vi "TargetNew.vi"() -> ()   [LabVIEW 2018]
uses:
  <vilib>/Platform/TimedLoop/XDataNode/timing_clust.ctl
  <vilib>/Platform/TimedLoop/XDataNode/nitl_modes.ctl
  <vilib>/Platform/TimedLoop/XDataNode/wakeup.ctl
  <vilib>/rvi/eio/common/nirviEmuTemplateMethod_errors.vi
  <vilib>/rvi/Emulation/niFpgaGetClockAttributes.vi
  <vilib>/rvi/Emulation/niFpgaSctlEmulationGetInTimedLoop.vi
  <vilib>/rvi/Emulation/niFpgaEmulationReportErrorSimple.vi
  <vilib>/rvi/Emulation/niFpgaCriticalErrorInLSC.vi
  <vilib>/rvi/interface/RandomDataEmulation/niFpgaRandomDataHandleErrors.vi
  <vilib>/rvi/Emulation/niFpgaProcessEmulError.vi
  <vilib>/eio/EIONode/EIONode.xnode
  <vilib>/Platform/TimedLoop/XDataNode/XDataNode.xnode
  <vilib>/rvi/DataTransferAndStorage/Container/XNode/niFpgaContainer.xnode
  <vilib>/rvi/interface/RandomDataEmulation/nirviRandomDataFpgaReadWriteTemplate.vi
  <vilib>/Platform/TimedLoop/XDataNode/XDNodeRunTimeDep.lvlib
panel:
  out "MISO 3":bool[](array[boolean])
  in  "10 2":u8=10
  out "out 2":bool
  out "out 2":u8
  out "out":u8
  out "out":bool
  in  "10":u8=10
  out "MISO 2":bool[](array[boolean])
  in  "Такт CSN 18":u8=18
  in  "Такт CSN 26":u8=26
  in  "26_STOP":u8=26
  in  "18_STOP":u8=18
  in  "18_R":u8=17
  in  "26_R":u8=25
  in  "17":u8=17
  in  "25":u8=25
  in  "TRIG":bool
  in  "Сброс индикатора":bool
  out "SPI_is_done":bool
  in  "Делитель 24/x":u8=2
  in  "Автомат":bool
  in  "RESET":bool
  in  "MOSI":bool[](array[boolean])=[FALSE, FALSE, FALSE, FALSE, FALSE, FALSE, FALSE, FALSE, FALSE, FALSE, FALSE, FALSE, FALSE, FALSE, FALSE, FALSE, FALSE, FALSE, FALSE, FALSE, FALSE, FALSE, FALSE, FALSE]
  in  "SPI":bool
  in  "8-bit(F)/16-bit(T)":bool
  in  "Stop_FPGA":bool
  # "0"
  # "0"
  # "7"
  # "7"
  # "Начало слова (8 bit)"
  # "Конец адреса (8 bit)"
  # "8"
  # "Начало адреса (8 bit)"
  # "14"
  # "15"
  # "R(F)/W(T) (8 bit)"
  # "Начало слова (16 bit)"
  # "15"
  # "Конец адреса (16 bit)"
  # "16"
  # "Начало адреса (16 bit)"
  # "22"
  # "R(F)/W(T) (16 bit)"
  # "23"
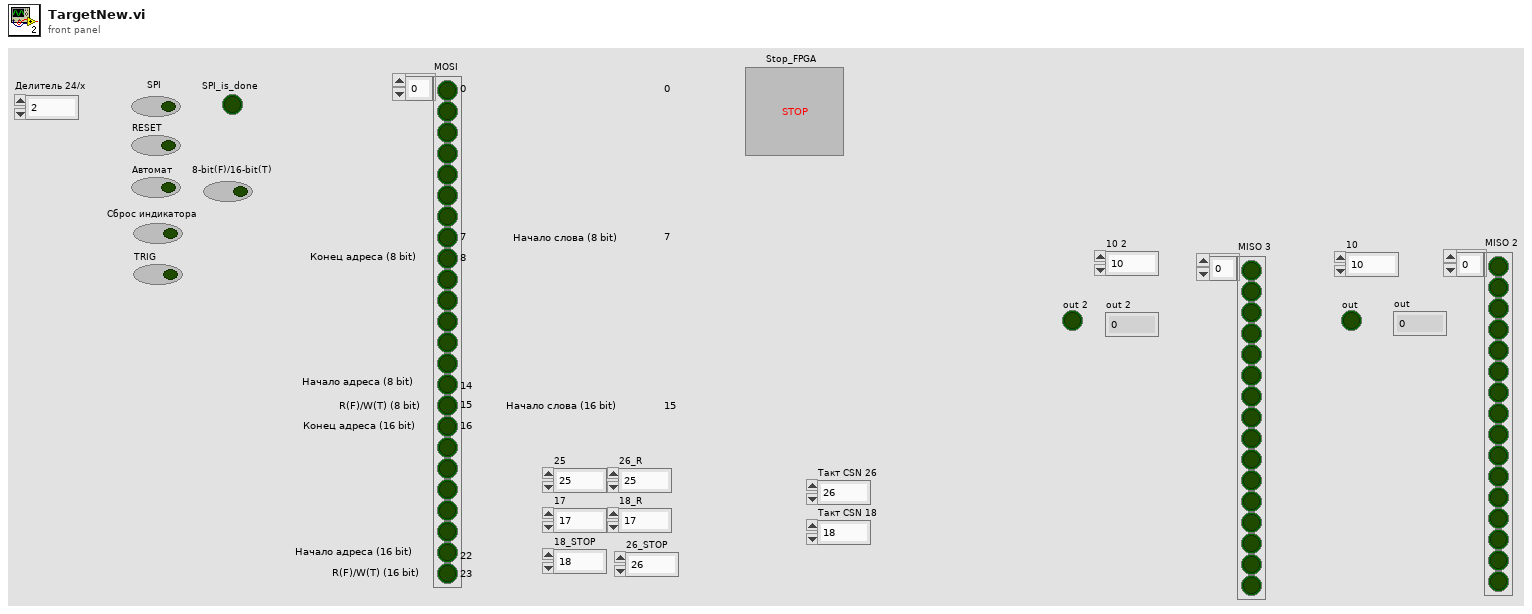
[diagram p1: front panel]
types:
  T1 = typedef "XDNodeRunTimeDep.lvlib/timing_clust.ctl" = cluster{"Expected End [f-1]":u64, "Actual End [f-1]":u64, "Finished Late? [f-1]":bool, "Expected End [i-1]":u64, "Actual End [i-1]":u64, "Finished Late? [i-1]":bool, "Expected Start [i]":u64, "Actual Start [i]":u64, "Expected Start [f]":u64, "Actual Start [f]":u64, "Source Name":string, "Structure Name":string, "Period":i64, "Deadline":i64, "Offset":i64, "Start":i64, "Priority":i32, "Timeout":i32, "Mode":T2, "Wakeup Reason":T3, "Error":errorcluster, "Source Type":string, "Secondary Source Type":string, "Global End Time":u64, "Global Start Time":u64, "Frame Duration":u64, "Iteration Duration":u64, "Assigned CPU":i32, "I/O Scan Engine Mode":u32}
  T2 = typedef "XDNodeRunTimeDep.lvlib/nitl_modes.ctl" = enum32{"No Change", "Process missed periods, maintain original phase", "Discard missed periods, maintain original phase", "Process missed periods, ignore original phase", "Discard missed periods, ignore original phase"}
  T3 = typedef "XDNodeRunTimeDep.lvlib/wakeup.ctl" = enum32{"Normal", "Aborted", "Asynchronous wakeup", "Timing source error", "Timed loop error", "Timeout"}
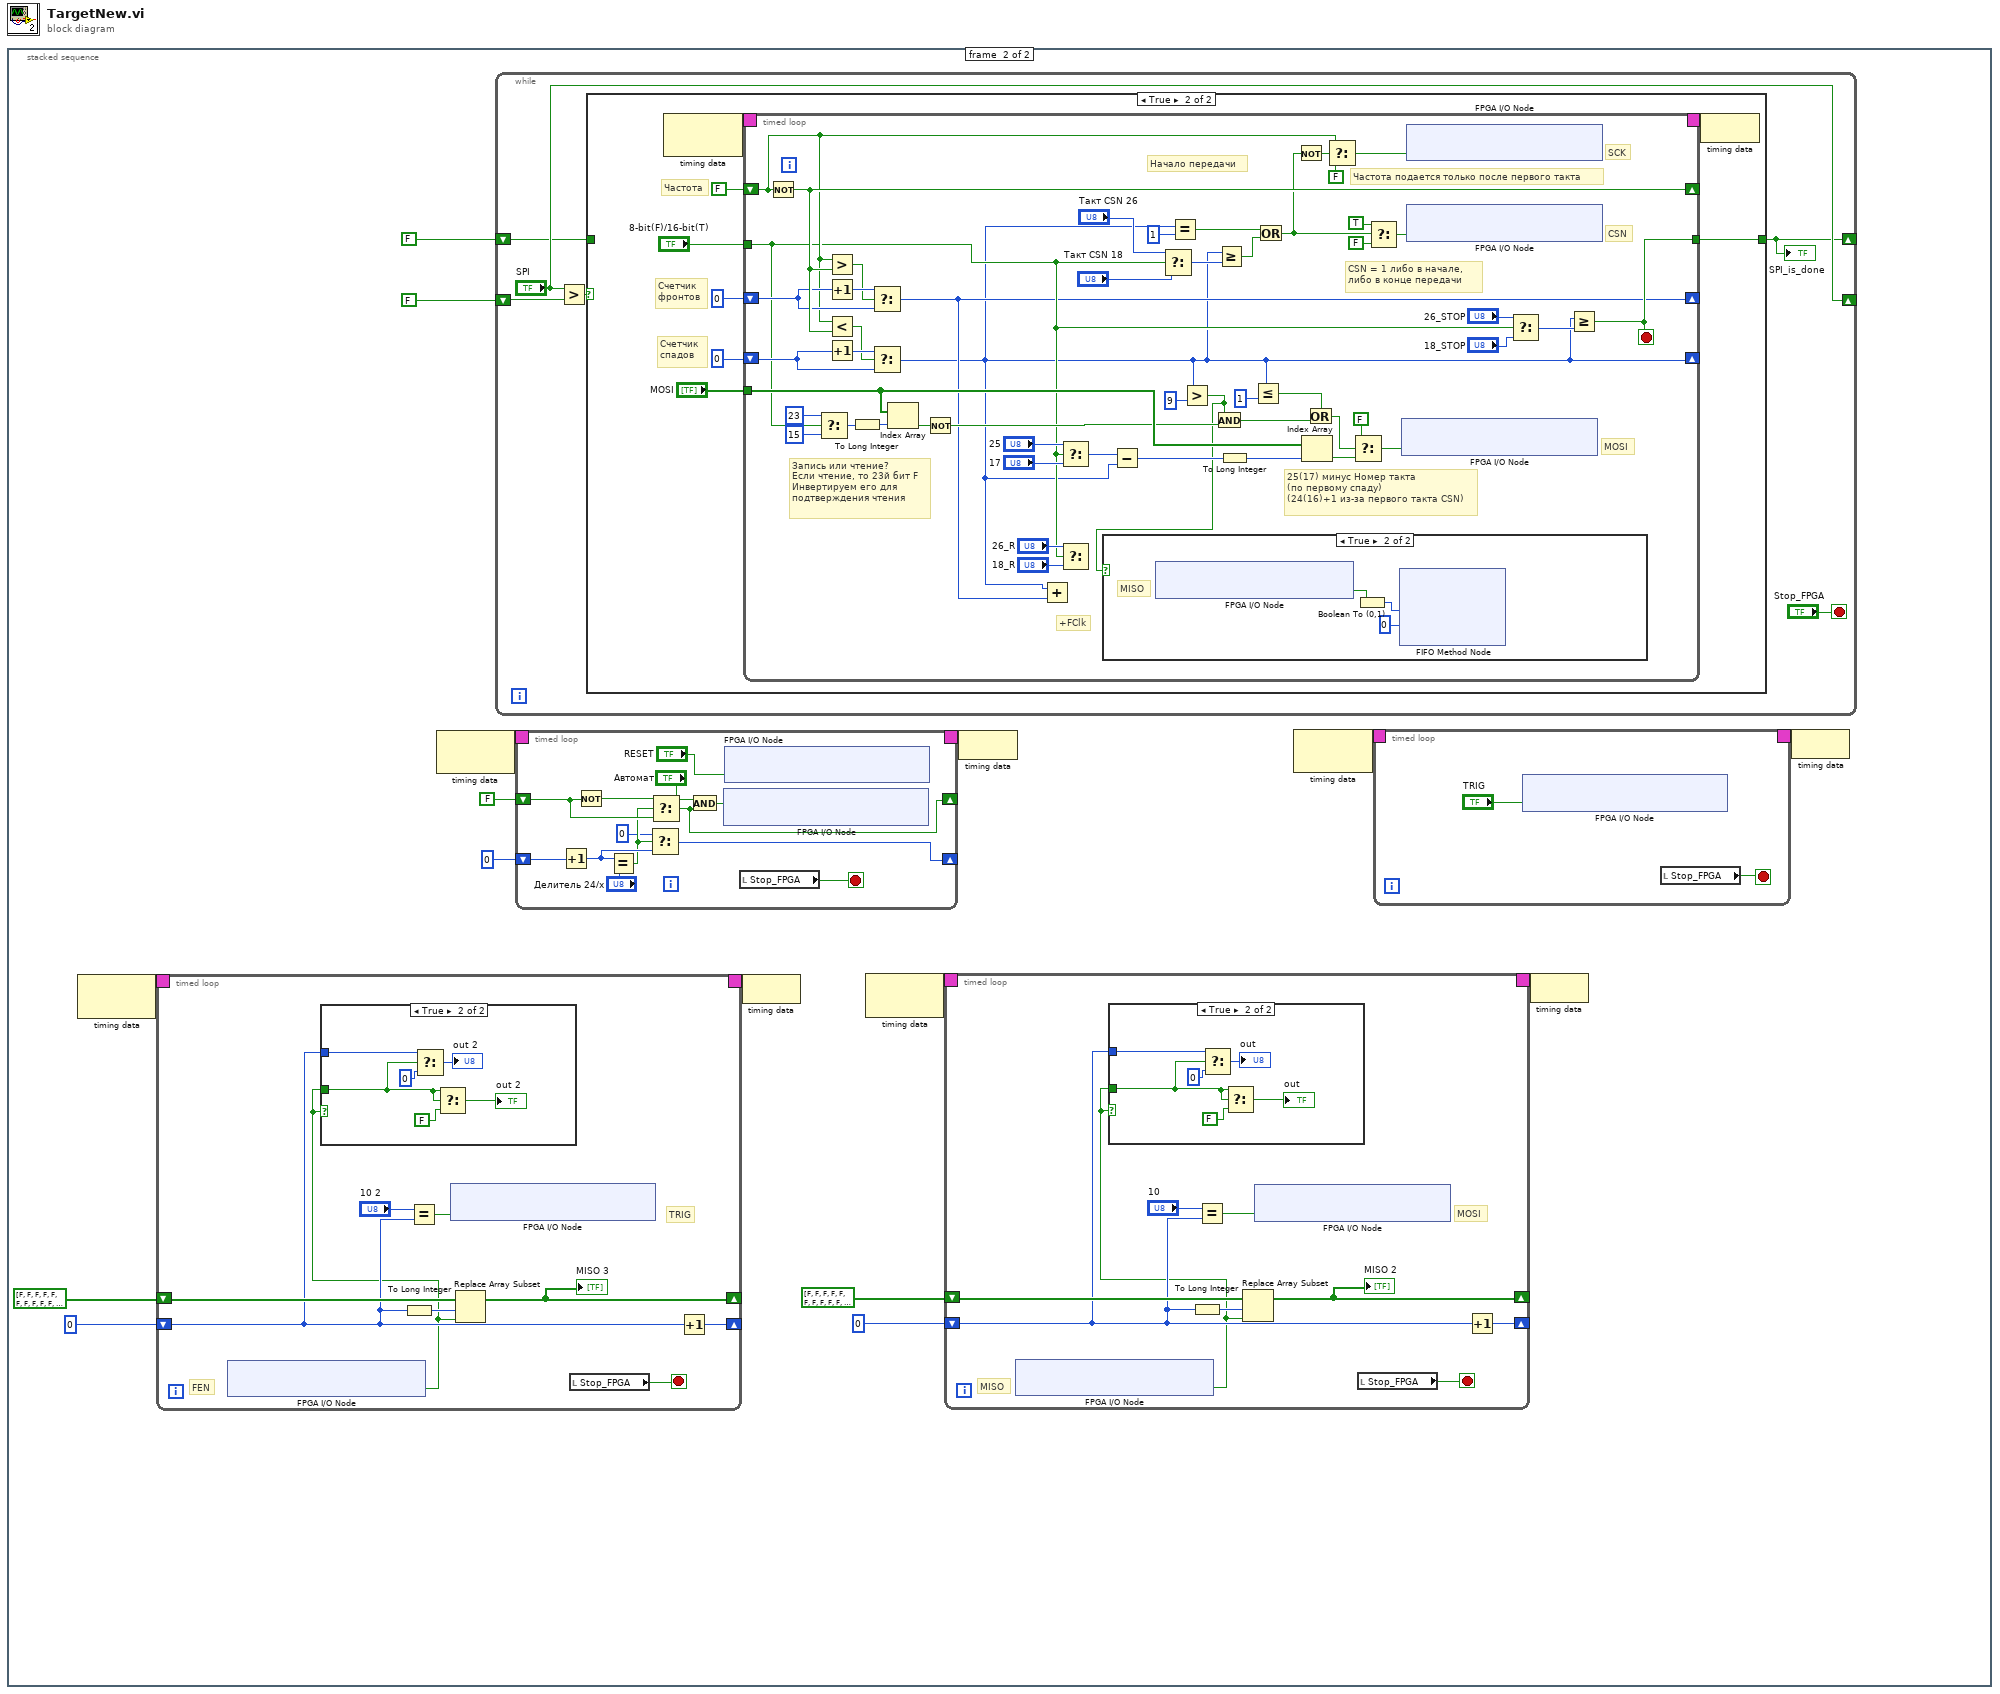
[diagram p0: block diagram]
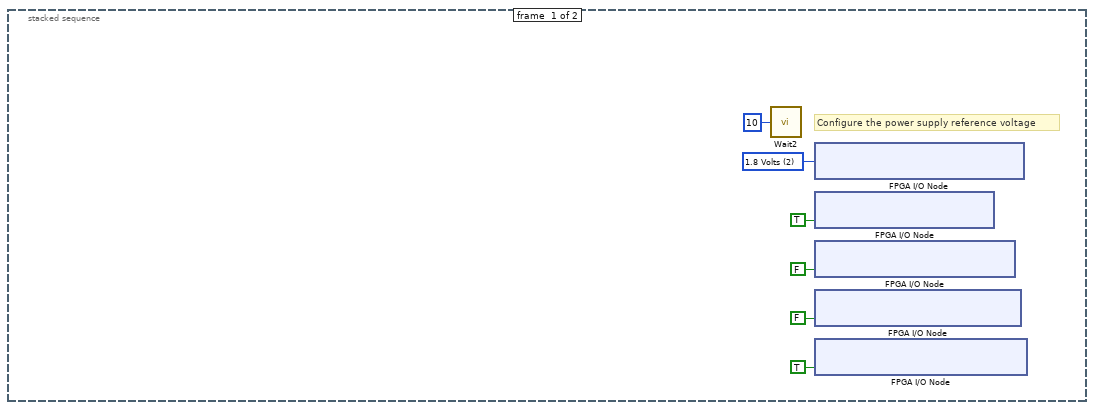
[diagram p2: hidden frame]
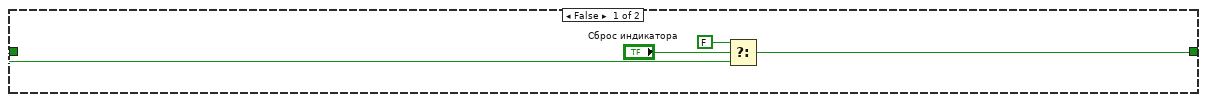
[diagram p5: hidden frame]
diagram:
  n1 = stacked-sequence {
    frame #0 {
      w6 = u8 2 items=["3.3 Volts", "2.5 Volts", "1.8 Volts"] ("Internal Power Supply Voltage")
      # "Configure the power supply reference voltage"
      n2 = call "Wait2"("Count(mSec)"=u8 10) -> ()  [unwired: 1 out]
      n3 = xnode "FPGA I/O Node"("IO Module\\Local_Supply_Select"=w6) -> ()  [unwired: 1 in, 1 out]
      n4 = xnode "FPGA I/O Node"("IO Module\\DDCA_PFI_WE"=TRUE ("IO Module\\DDCB_PFI_WE")) -> ()  [unwired: 1 in, 1 out]
      n5 = xnode "FPGA I/O Node"("IO Module\\DDCA_DIO0-7_WE"=FALSE ("IO Module\\DDCA_DIO0-7_WE")) -> ()  [unwired: 1 in, 1 out]
      n6 = xnode "FPGA I/O Node"("IO Module\\DDCA_DIO8-15_WE"=FALSE ("IO Module\\DDCA_DIO8-15_WE")) -> ()  [unwired: 1 in, 1 out]
      n7 = xnode "FPGA I/O Node"("IO Module\\DDCA_DIO16-23_WE"=TRUE ("IO Module\\DDCA_DIO16-23_WE")) -> ()  [unwired: 1 in, 1 out]
    }
    frame #1 {
      n8 = node-c288() -> (w10:T1)  [unwired: 1 in]
      n9 = timed-loop {
        timing: w10 -> [_]
        timing-out: [_] -> w9
        shift-right: [w30] -> _
        shift-left: bool[] [FALSE, FALSE, FALSE, FALSE, FALSE, FALSE, FALSE, FALSE, FALSE, FALSE, FALSE, FALSE, FALSE, FALSE, FALSE, FALSE] -> [w26]
        shift-right: [w27] -> _
        shift-left: u8 0 -> [w25]
        stop <- w28 stop-if-true
        # "FEN"
        # "TRIG"
        n10 = xnode "FPGA I/O Node"() -> ("IO Module\\DDCA_DIO1_Read"=w24:bool)  [unwired: 1 in, 1 out]
        n11 = case shown="True" w24 {
          tunnel: w25 -> [_ w33]
          tunnel: w24 -> [_ w32]
          frame False {
          }
          frame True {
            n12 = Select(t=w33, s=w32, f=u8 0) -> (s? t:f=→"out 2":u8)
            n13 = Select(t=w32, s=w32, f=FALSE ("t")) -> (s? t:f=→"out 2":bool)
          }
        }
        n14 = To Long Integer(number=w25) -> (32bit integer=w31:i32)
        n15 = Equal?(x="10 2", y=w25) -> (x = y?=w23:bool)
        n16 = xnode "FPGA I/O Node"("IO Module\\DDCA_DIO18_Write"=w23) -> ()  [unwired: 1 in, 1 out]
        n17 = Replace Array Subset(array=w26, new element=w24, index=w31) -> (w30:bool[])
        "MISO 3" <- w30
        n18 = local read "Stop_FPGA"() -> (w28:bool)
        n19 = Increment(x=w25) -> (x+1=w27:u8)
      }
      n20 = node-c288() -> (w21:T1)  [unwired: 1 in]
      n21 = while {
        shift-right: ["SPI"] -> _
        shift-left: FALSE -> [w89]
        shift-right: [w84] -> _
        shift-left: FALSE -> [w85]
        stop <- "Stop_FPGA" stop-if-true
        n22 = Greater?(x="SPI", y=w89) -> (0:w88:bool)
        n23 = case shown="True" w88 {
          tunnel: [w92 w96] -> w84
          tunnel: w85 -> [w90 _]
          frame False {
            n24 = Select(t=FALSE, s="Сброс индикатора", f=w90) -> (s? t:f=w92:bool)
          }
          frame True {
            # "Счетчик\nфронтов"
            # "Счетчик\nспадов"
            # "Частота"
            n25 = node-c288() -> (w101:T1)  [unwired: 1 in]
            n26 = timed-loop {
              timing: w101 -> [_]
              timing-out: [_] -> w100
              shift-right: [w105] -> _
              shift-left: u8 0 -> [w148]
              shift-right: [w151] -> _
              shift-left: FALSE -> [w142]
              shift-right: [w104] -> _
              shift-left: u8 0 -> [w149]
              tunnel: [w110] -> w96
              tunnel: "8-bit(F)/16-bit(T)" -> [w107]
              tunnel: "MOSI" -> [w129]
              stop <- w110 stop-if-true
              # "+FClk"
              # "MOSI"
              # "25(17) минус Номер такта\n(по первому спаду)\n(24(16)+1 из-за первого такта CSN)"
              # "Запись или чтение?\nЕсли чтение, то 23й бит F\nИнвертируем его для\nподтверждения чтения"
              # "Начало передачи"
              # "CSN"
              # "Частота подается только после первого такта"
              # "CSN = 1 либо в начале,\nлибо в конце передачи"
              # "SCK"
              n27 = Not(x=w142) -> (.not. x?=w151:bool)
              n28 = Select(t=u8 23, s=w107, f=u8 15) -> (s? t:f=w139:u8)
              n29 = Greater?(x=w142, y=w151) -> (0:w114:bool)
              n30 = Increment(x=w148) -> (x+1=w152:u8)
              n31 = Less?(x=w142, y=w151) -> (x < y?=w123:bool)
              n32 = Increment(x=w149) -> (x+1=w150:u8)
              n33 = To Long Integer(number=w139) -> (32bit integer=w138:i32)
              n34 = Select(t=w152, s=w114, f=w148) -> (s? t:f=w105:u8)
              n35 = Select(t=w150, s=w123, f=w149) -> (s? t:f=w104:u8)
              n36 = Index Array(array=w129, index=w138) -> (element=w124:bool)
              n37 = Not(x=w124) -> (.not. x?=w122:bool)
              n38 = Add(x=w104, y=w105) -> ()  [unwired: 1 out]
              n39 = Select(t="25", s=w107, f="17") -> (s? t:f=w119:u8)
              n40 = Select(t="26_R", s=w107, f="18_R") -> ()  [unwired: 1 out]
              n41 = Subtract(x=w119, y=w104) -> (x-y=w113:u8)
              n42 = Select(t="Такт CSN 26", s=w107, f="Такт CSN 18") -> (s? t:f=w118:u8)
              n43 = Equal?(x=w104, y=u8 1 ("1")) -> (x = y?=w144:bool)
              n44 = Greater?(x=w104, y=u8 9 ("18")) -> (0:w102:bool)
              n45 = case shown="True" w102 {
                frame False {
                }
                frame True {
                  # "MISO"
                  n46 = xnode "FPGA I/O Node"() -> ("IO Module\\DDCA_DIO0_Read"=w155:bool)  [unwired: 1 in, 1 out]
                  n47 = Boolean To (0,1)(Boolean=w155) -> (0, 1=w154:i16)
                  n48 = xnode ("FIFO Method Node")("Element"=w154, "Timeout"=0) -> ()  [unwired: 1 in, 2 out]
                }
              }
              n49 = And(x=w102, y=w122) -> (x .and. y?=w133:bool)
              n50 = Greater Or Equal?(x=w104, y=w118) -> (x >= y?=w115:bool)
              n51 = To Long Integer(number=w113) -> (32bit integer=w147:i32)
              n52 = Less Or Equal?(x=w104, y=u8 1 ("18")) -> (x <= y?=w131:bool)
              n53 = Or(x=w144, y=w115) -> (x .or. y?=w116:bool)
              n54 = Not(x=w116) -> (.not. x?=w117:bool)
              n55 = Index Array(array=w129, index=w147) -> (element=w137:bool)
              n56 = Or(x=w131, y=w133) -> (x .or. y?=w132:bool)
              n57 = Select(t=w142, s=w117, f=FALSE) -> (s? t:f=w143:bool)
              n58 = Select(t=FALSE, s=w132, f=w137) -> (s? t:f=w103:bool)
              n59 = Select(t=TRUE, s=w116, f=FALSE) -> (s? t:f=w135:bool)
              n60 = xnode "FPGA I/O Node"("IO Module\\DDCA_PFI3_Write"=w103) -> ()  [unwired: 1 in, 1 out]
              n61 = xnode "FPGA I/O Node"("IO Module\\DDCA_PFI1_Write"=w143) -> ()  [unwired: 1 in, 1 out]
              n62 = xnode "FPGA I/O Node"("IO Module\\DDCA_PFI2_Write"=w135) -> ()  [unwired: 1 in, 1 out]
              n63 = Select(t="26_STOP", s=w107, f="18_STOP") -> (s? t:f=w106:u8)
              n64 = Greater Or Equal?(x=w104, y=w106) -> (x >= y?=w110:bool)
            }
            n65 = node-c288(w100) -> ()
          }
        }
        "SPI_is_done" <- w84
      }
      n66 = timed-loop {
        timing: w21 -> [_]
        timing-out: [_] -> w20
        shift-right: [w68] -> _
        shift-left: FALSE -> [w77]
        shift-right: [w69] -> _
        shift-left: u8 0 -> [w74]
        stop <- w67 stop-if-true
        n67 = Increment(x=w74) -> (x+1=w72:u8)
        n68 = Not(x=w77) -> (.not. x?=w78:bool)
        n69 = Equal?(x=w72, y="Делитель 24/x") -> (x = y?=w71:bool)
        n70 = Select(t=u8 0, s=w71, f=w72) -> (s? t:f=w69:u8)
        n71 = Select(t=w78, s=w71, f=w77) -> (s? t:f=w68:bool)
        n72 = And(x="Автомат", y=w68) -> (x .and. y?=w76:bool)
        n73 = xnode "FPGA I/O Node"("IO Module\\DDCA_DIO16_Write"=w76) -> ()  [unwired: 1 in, 1 out]
        n74 = xnode "FPGA I/O Node"("IO Module\\DDCA_DIO19_Write"="RESET") -> ()  [unwired: 1 in, 1 out]
        n75 = local read "Stop_FPGA"() -> (w67:bool)
      }
      n76 = node-c288(w9) -> ()
      n77 = node-c288() -> (w14:T1)  [unwired: 1 in]
      n78 = timed-loop {
        timing: w14 -> [_]
        timing-out: [_] -> w13
        shift-right: [w49] -> _
        shift-left: bool[] [FALSE, FALSE, FALSE, FALSE, FALSE, FALSE, FALSE, FALSE, FALSE, FALSE, FALSE, FALSE, FALSE, FALSE, FALSE, FALSE] -> [w44]
        shift-right: [w45] -> _
        shift-left: u8 0 -> [w43]
        stop <- w46 stop-if-true
        # "MISO"
        # "MOSI"
        n79 = xnode "FPGA I/O Node"() -> ("IO Module\\DDCA_DIO0_Read"=w42:bool)  [unwired: 1 in, 1 out]
        n80 = case shown="True" w42 {
          tunnel: w43 -> [_ w52]
          tunnel: w42 -> [_ w51]
          frame False {
          }
          frame True {
            n81 = Select(t=w52, s=w51, f=u8 0) -> (s? t:f=→"out":u8)
            n82 = Select(t=w51, s=w51, f=FALSE ("t")) -> (s? t:f=→"out":bool)
          }
        }
        n83 = To Long Integer(number=w43) -> (32bit integer=w50:i32)
        n84 = Equal?(x="10", y=w43) -> (x = y?=w48:bool)
        n85 = Replace Array Subset(array=w44, new element=w42, index=w50) -> (w49:bool[])
        "MISO 2" <- w49
        n86 = xnode "FPGA I/O Node"("IO Module\\DDCA_PFI3_Write"=w48) -> ()  [unwired: 1 in, 1 out]
        n87 = local read "Stop_FPGA"() -> (w46:bool)
        n88 = Increment(x=w43) -> (x+1=w45:u8)
      }
      n89 = node-c288(w20) -> ()
      n90 = node-c288() -> (w16:T1)  [unwired: 1 in]
      n91 = timed-loop {
        timing: w16 -> [_]
        timing-out: [_] -> w15
        stop <- w61 stop-if-true
        n92 = xnode "FPGA I/O Node"("IO Module\\DDCA_DIO18_Write"="TRIG") -> ()  [unwired: 1 in, 1 out]
        n93 = local read "Stop_FPGA"() -> (w61:bool)
      }
      n94 = node-c288(w13) -> ()
      n95 = node-c288(w15) -> ()
    }
  }
